vi "PQLaserDriver.vi"() -> ()   [LabVIEW 2020]
panel:
  in  "preselection product":enum8{"only Sepia II", "only Solea", "all"}(ring)=enum."all" caption="Select product type"
  out "Deviceinfo (TXT)":string
  out "error out":errorcluster caption="Error OUT"
  in  "StayOpen":bool caption="On Stop stay open"
  out "VI_Cnt":i32
  in  "Stop button":bool
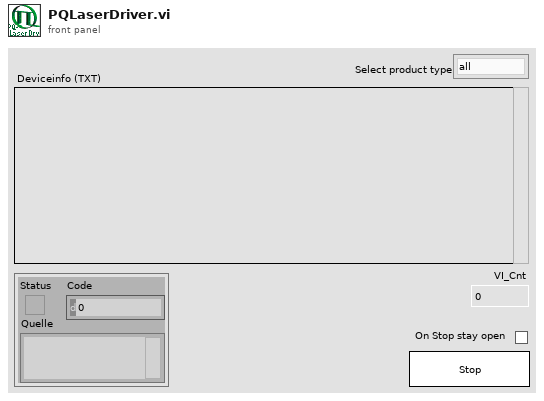
[diagram p1: front panel]
types:
  T1 = cluster{"left":i16, "top":i16, "right":i16, "bottom":i16}
  T2 = cluster{"LibVersion":string, "USB-Port":i32, "ProductModel":string, "SerialNumber":string, "Descriptor":string, "Slots":cluster{"SlotId":i32, "IsPrimary":u8, "IsBackPlane":u8, "HasUptimeCounter":u8, "ModulTypeAbbr":string, "SerialNumber":string, "HasSecondary":i32}[]}
  T3 = cluster{"SlotId":i32, "IsPrimary":u8, "IsBackPlane":u8, "HasUptimeCounter":u8, "ModulTypeAbbr":string, "SerialNumber":string, "HasSecondary":i32}[]
  T4 = typedef "LVRectTypeDef.ctl" = cluster{"Left":i16, "Top":i16, "Right":i16, "Bottom":i16}
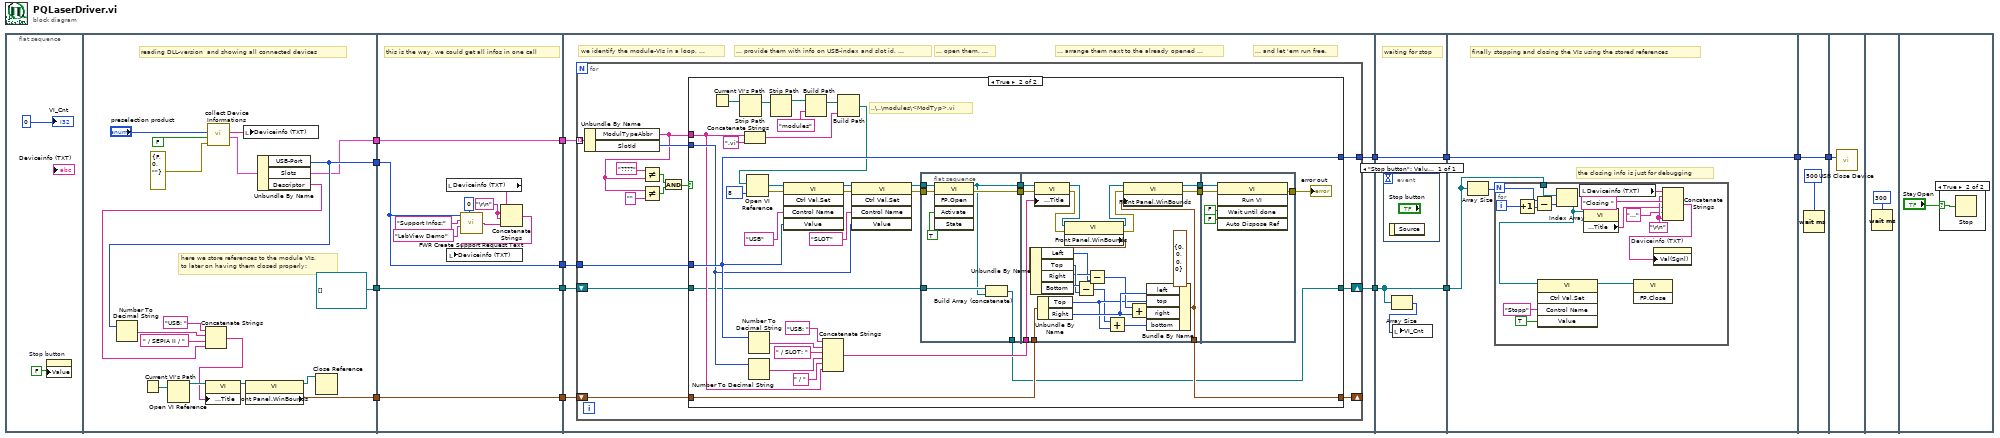
[diagram p0: block diagram]
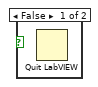
[diagram p3: hidden frame]
diagram:
  n1 = flat-sequence {
    tunnel: [w20] -> w10
    tunnel: [w19] -> w8
    tunnel: [refnum<vi>[] [] ("RefArr")] -> w5
    tunnel: [w18] -> w3
    tunnel: w10 -> [w44]
    tunnel: [w44] -> w9
    tunnel: w8 -> [w39]
    tunnel: [w39] -> w7
    tunnel: [w38] -> w6
    tunnel: w5 -> [w38]
    tunnel: [w37] -> w4
    tunnel: w3 -> [w37]
    tunnel: [w51] -> w13
    tunnel: w9 -> [w50]
    tunnel: w7 -> [w49]
    tunnel: w6 -> [w48]
    tunnel: w4 -> [w47]
    tunnel: [w46] -> w1
    tunnel: [w141] -> w14
    tunnel: w13 -> [w141]
    tunnel: [w140] -> w2
    tunnel: w1 -> [w140]
    tunnel: [w144] -> w12
    tunnel: w14 -> [w144]
    tunnel: w2 -> [w142]
    tunnel: w12 -> [w161]
    tunnel: [w161] -> w11
    tunnel: w11 -> [w162]
    frame #0 {
      n2 = property on="Stop button" class="Bool (strict)"("Value"=FALSE ("Stop button")) -> ()  [unwired: 2 in, 2 out]
      "VI_Cnt" <- 0 ("VI_Cnt")
    }
    frame #1 {
      # "here we store references to the module VIs,\nto later on having them closed properly:"
      # "reading DLL-version  and showing all connected devices"
      n3 = Current VI's Path() -> (path=w25:path)
      n4 = Open VI Reference(vi path=w25) -> (vi reference=w30:refnum<vi>)  [unwired: 5 in, 1 out]
      n5 = call "collect Device Informations.vi"("error in (no error)"=errorcluster {"status"=FALSE, "code"=0, "source"=""}, "close device?"=FALSE, "preselection product"="preselection product") -> ("device infos"=w21:T2, "Deviceinfo (TXT)"=w34:string)  [unwired: 1 in, 2 out]
      n6 = local write "Deviceinfo (TXT)"(w34) -> ()
      n7 = Unbundle By Name(w21) -> ("USB-Port"=w20:i32, "Slots"=w19:T3, "Descriptor"=w32:string)
      n8 = Number To Decimal String(number=w20) -> (decimal integer string=w28:string)  [unwired: 1 in]
      n9 = Concatenate Strings("USB: " ("Front Panel Window:Title"), w28, " / SEPIA II / " ("string"), w32) -> (w26:string)
      n10 = property class="VI"(reference=w30, "Front Panel.Title"=w26) -> (reference out=w31:refnum<vi>)  [unwired: 1 in, 1 out]
      n11 = property class="VI"(reference=w31) -> (reference out=w24:refnum<vi>, "Front Panel.WinBounds"=w18:T4)  [unwired: 1 in, 1 out]
      n12 = Close Reference(reference=w24) -> ()  [unwired: 1 in, 1 out]
    }
    frame #2 {
      w35 = "\r\n"
      # "this is the way, we could get all infos in one call"
      n13 = local read "Deviceinfo (TXT)"() -> (w43:string)
      n14 = call "FWR Create Support Request Text.vi"("DevIdx"=w44, "Preamble"="Support Infos:", "CallingSW"="LabView Demo", "Options"=0) -> ("SupportRequestText"=w36:string)  [unwired: 1 in, 2 out]
      n15 = Concatenate Strings(w43, w35, w35, w36) -> (w42:string)
      n16 = local write "Deviceinfo (TXT)"(w42) -> ()
    }
    frame #3 {
      # "... open them, ..."
      # "... provide them with info on USB-index and slot id, ..."
      # "... and let 'em run free."
      # "... arrange them next to the already opened ..."
      # "we identify the module-VIs in a loop, ..."
      n17 = for {
        tunnel: w49 -> [w65] mode=indexing
        tunnel: w50 -> [w62]
        tunnel: [w57] -> w51
        shift-right: [w55] -> _
        shift-left: w47 -> [w56]
        shift-right: [w52] -> w46
        shift-left: w48 -> [w54]
        n18 = Unbundle By Name(w65) -> ("ModulTypeAbbr"=w53:string, "SlotId"=w63:i32)
        n19 = Not Equal?(x=w53, y="") -> (x != y?=w59:bool)
        n20 = Not Equal?(x="????", y=w53) -> (x != y?=w60:bool)
        n21 = And(x=w60, y=w59) -> (x .and. y?=w58:bool)
        n22 = case shown="True" w58 {
          tunnel: w53 -> [_ w83]
          tunnel: w63 -> [_ w84]
          tunnel: w62 -> [w67 w85]
          tunnel: [w67 w85] -> w57
          tunnel: w56 -> [w68 w73]
          tunnel: [w68 w74] -> w55
          tunnel: w54 -> [w66 w72]
          tunnel: [w66 w71] -> w52
          frame False {
          }
          frame True {
            # "..\\..\\modules\\<ModTyp>.vi"
            n23 = Current VI's Path() -> (path=w102:path)
            n24 = Strip Path(path=w102) -> (stripped path=w101:path)  [unwired: 1 out]
            n25 = Concatenate Strings(w83, ".vi" ("string")) -> (w97:string)
            n26 = Number To Decimal String(number=w85) -> (decimal integer string=w89:string)  [unwired: 1 in]
            n27 = Number To Decimal String(number=w84) -> (decimal integer string=w87:string)  [unwired: 1 in]
            n28 = Strip Path(path=w101) -> (stripped path=w100:path)  [unwired: 1 out]
            n29 = Build Path(base path=w100, name or relative path="modules") -> (appended path=w99:path)
            n30 = Concatenate Strings("USB: " ("Front Panel Window:Title"), w89, " / SLOT: " ("string"), w87, " / " ("string"), w83) -> (w75:string)
            n31 = Build Path(base path=w99, name or relative path=w97) -> (appended path=w82:path)
            n32 = Open VI Reference(vi path=w82, options=8) -> (vi reference=w96:refnum<vi>, error out=w95:errorcluster)  [unwired: 4 in]
            n33 = invoke class="VI" method="Ctrl Val.Set"(reference=w96, error in=w95, "Control Name"="USB", "Value"=w85) -> (reference out=w93:refnum<vi>, error out=w92:errorcluster)  [unwired: 1 in, 3 out]
            n34 = invoke class="VI" method="Ctrl Val.Set"(reference=w93, error in=w92, "Control Name"="SLOT", "Value"=w84) -> (reference out=w80:refnum<vi>, error out=w79:errorcluster)  [unwired: 1 in, 3 out]
            n35 = flat-sequence {
              tunnel: [w105] -> w70
              tunnel: [w109] -> w69
              tunnel: w80 -> [w108]
              tunnel: w79 -> [w107]
              tunnel: w72 -> [w106]
              tunnel: [w104] -> w71
              tunnel: w70 -> [w132]
              tunnel: [w126] -> w77
              tunnel: w69 -> [w131]
              tunnel: [w125] -> w76
              tunnel: w75 -> [w133]
              tunnel: [w122] -> w74
              tunnel: w73 -> [w111]
              tunnel: w77 -> [w137]
              tunnel: w76 -> [w136]
              tunnel: [w135] -> w78
              frame #0 {
                n36 = invoke class="VI" method="FP.Open"(reference=w108, error in=w107, "Activate"=TRUE ("Activate?")) -> (reference out=w105:refnum<vi>, error out=w109:errorcluster)  [unwired: 2 in, 3 out]
                n37 = Build Array (concatenate)(w106, w105) -> (w104:refnum<vi>[])
              }
              frame #1 {
                n38 = property class="VI"(reference=w132, error in=w131, "Front Panel.Title"=w133) -> (reference out=w129:refnum<vi>, error out=w130:errorcluster)
                n39 = Unbundle By Name(w111) -> ("Top"=w113:i16, "Right"=w115:i16)
                n40 = property class="VI"(reference=w129, error in=w130) -> (reference out=w128:refnum<vi>, error out=w127:errorcluster, "Front Panel.WinBounds"=w124:T4)
                n41 = Unbundle By Name(w124) -> ("Left"=w118:i16, "Top"=w120:i16, "Right"=w119:i16, "Bottom"=w121:i16)
                n42 = Subtract(x=w121, y=w120) -> (x-y=w112:i16)
                n43 = Subtract(x=w119, y=w118) -> (x-y=w114:i16)
                n44 = Add(x=w112, y=w113) -> (x+y=w117:i16)
                n45 = Add(x=w114, y=w115) -> (x+y=w116:i16)
                n46 = Bundle By Name(cluster=T1 {"left"=0, "top"=0, "right"=0, "bottom"=0} ("Front Panel Window:Window Bounds"), "left"=w115, "top"=w113, "right"=w116, "bottom"=w117) -> (w122:T1)
                n47 = property class="VI"(reference=w128, error in=w127, "Front Panel.WinBounds"=w122) -> (reference out=w126:refnum<vi>, error out=w125:errorcluster)
              }
              frame #2 {
                n48 = invoke class="VI" method="Run VI"(reference=w137, error in=w136, "Wait until done"=FALSE ("Wait Until Done"), "Auto Dispose Ref"=FALSE ("Wait Until Done")) -> (error out=w135:errorcluster)  [unwired: 1 in, 4 out]
              }
            }
            "error out" <- w78
          }
        }
      }
    }
    frame #4 {
      # "waiting for stop"
      n49 = event shown="[0] \"Stop button\": Value Change" {
        selector: _ -> [_]
        dyn-events: _ -> [_]
        timeout: _ -> [_]
        event "Stop button": Value Change {
          n50 = event-data() -> ()  [unwired: 1 in, 1 out]
        }
      }
      n51 = Array Size(array=w140) -> (size(s)=w139:i32)
      n52 = local write "VI_Cnt"(w139) -> ()
    }
    frame #5 {
      # "the closing info is just for debugging"
      # "finally stopping and closing the VIs using the stored references"
      n53 = Array Size(array=w142) -> (size(s)=w143:i32)
      n54 = for {
        N: w143 -> [w157]
        tunnel: w142 -> [w159]
        i -> [w156]
        w151 = "\r\n"
        n55 = Increment(x=w156) -> (x+1=w155:i32)
        n56 = Subtract(x=w157, y=w155) -> (x-y=w158:i32)
        n57 = Index Array(array=w159, index=w158) -> (element=w154:refnum<vi>)
        n58 = invoke class="VI" method="Ctrl Val.Set"(reference=w154, "Control Name"="Stopp", "Value"=TRUE) -> (reference out=w147:refnum<vi>)  [unwired: 2 in, 4 out]
        n59 = local read "Deviceinfo (TXT)"() -> (w153:string)
        n60 = property class="VI"(reference=w154) -> ("Front Panel.Title"=w150:string)  [unwired: 1 in, 2 out]
        n61 = invoke class="VI" method="FP.Close"(reference=w147) -> ()  [unwired: 2 in, 3 out]
        n62 = Concatenate Strings(w153, w151, "Closing ", w150, "...", w151) -> (w148:string)
        n63 = property on="Deviceinfo (TXT)" class="Str"("Val(Sgnl)"=w148) -> ()  [unwired: 2 in, 2 out]
      }
    }
    frame #6 {
      n64 = Wait (ms)(milliseconds to wait=u32 500) -> ()  [unwired: 1 out]
    }
    frame #7 {
      n65 = call "USB Close Device.vi"("DevIdx"=w162) -> ()  [unwired: 1 in, 1 out]
    }
    frame #8 {
      n66 = Wait (ms)(milliseconds to wait=u32 300) -> ()  [unwired: 1 out]
    }
    frame #9 {
      n67 = case shown="True" "StayOpen" {
        selector: "StayOpen" -> [_ w165]
        frame False {
          n68 = Quit LabVIEW() -> ()  [unwired: 1 in]
        }
        frame True {
          n69 = Stop(stop? (T)=w165) -> ()
        }
      }
    }
  }
